vi "ddetest.vi"() -> ()   [LabVIEW 2016]
panel:
  in  "stop":bool
  out "data read":string
  in  "read item":string="double1"
  in  "write value":string="4.1"
  in  "write item":string="double1"
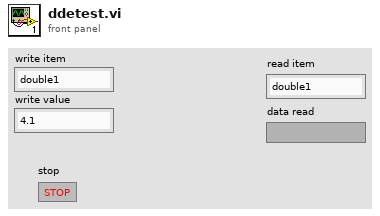
[diagram p1: front panel]
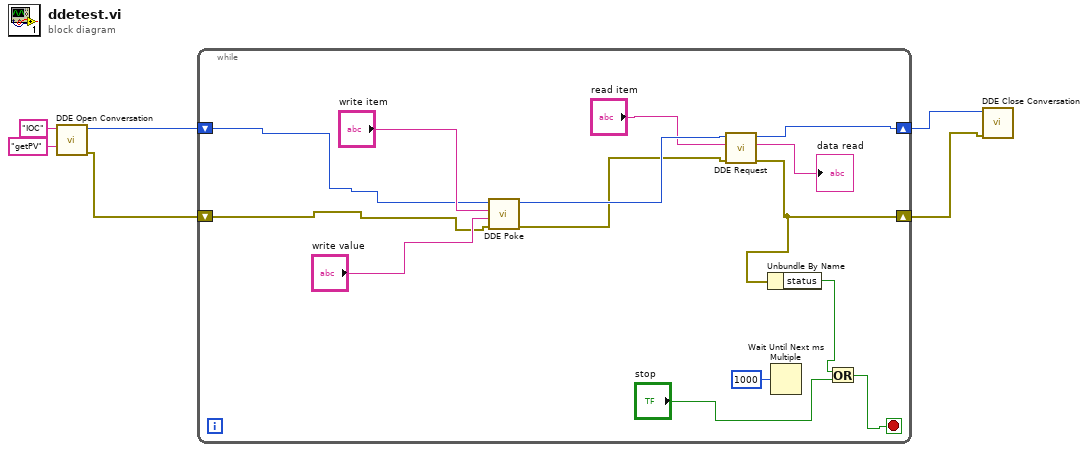
[diagram p0: block diagram]
diagram:
  n1 = call <vilib>:"DDE Open Conversation.vi"("topic"="getPV", "service"="IOC") -> ("error out"=w3:errorcluster, "conversation refnum"=w4:u32)  [unwired: 6 in]
  n2 = while {
    shift-right: [w10] -> w1
    shift-left: w3 -> [w12]
    shift-right: [w11] -> w2
    shift-left: w4 -> [w13]
    stop <- w7 stop-if-true
    n3 = call <vilib>:"DDE Poke.vi"("error in (no error)"=w12, "data"="write value", "item"="write item", "conversation refnum in"=w13) -> ("error out"=w15:errorcluster, "conversation refnum out"=w17:u32)  [unwired: 4 in]
    n4 = call <vilib>:"DDE Request.vi"("error in (no error)"=w15, "item"="read item", "conversation refnum in"=w17) -> ("error out"=w10:errorcluster, "data"=→"data read":string, "conversation refnum out"=w11:u32)  [unwired: 4 in]
    n5 = Unbundle By Name(w10) -> ("status"=w8:bool)
    n6 = Wait Until Next ms Multiple(millisecond multiple=u32 1000) -> ()  [unwired: 1 out]
    n7 = Or(x=w8, y="stop") -> (x .or. y?=w7:bool)
  }
  n8 = call <vilib>:"DDE Close Conversation.vi"("error in (no error)"=w1, "conversation refnum"=w2) -> ()  [unwired: 7 in, 1 out]
